vi "Test Initialization.vi"() -> ()   [LabVIEW 2020]
uses:
  Typedefs/FABR-Parameters.ctl
  Typedefs/FABR-Stimulus.ctl
  Typedefs/FABR-Sequence.ctl
  Typedefs/FABR-Order.ctl
  Typedefs/FABR-Response.ctl
  Typedefs/FABR-Runtime Data.ctl
  Typedefs/FABR-Stimulus Ticket.ctl
  Typedefs/FABR-Stimulus Condition.ctl
panel:
  out "resps":T1[](array[typedef])
  out "size(s)":i32
  out "stims":T1[](array[typedef])
  out "Tones":dbl[][](graph)
  out "SCL":cluster{T2[]}[](array[cluster])
  out "Runtime":T3
  in  "Params":T4={"Stimulus"={"Destination"="Speaker", "Rep rate (/sec)"=50.0, "Alternate Polarity"=FALSE, "Duration (ms)"=5.0, "Ramp (ms)"=0.5, "Fs (Hz)"=100000.0, "Frame size (s)"=1.0}, "Sequence"={"Freq"={"Start (kHz)"=0.25, "Stop (kHz)"=4.0, "Step (oct)"=1.0, "Skip (oct)"=2.0}, "Level"={"Start (dB)"=20, "Stop (dB)"=80, "Step (dB)"=10}, "Order"=enum."Interleaved"}, "Response"={"Gain"=1.0, "Averages"=0, "Window (ms)"=0.0, "Fs (Hz)"=25000.0}, "Reject"=0.0} {"Sequence"."Level"."Start (dB)" step=5; "Sequence"."Freq"."Start (kHz)" step=5.0; "Response"."Window (ms)" format="%.2f"}
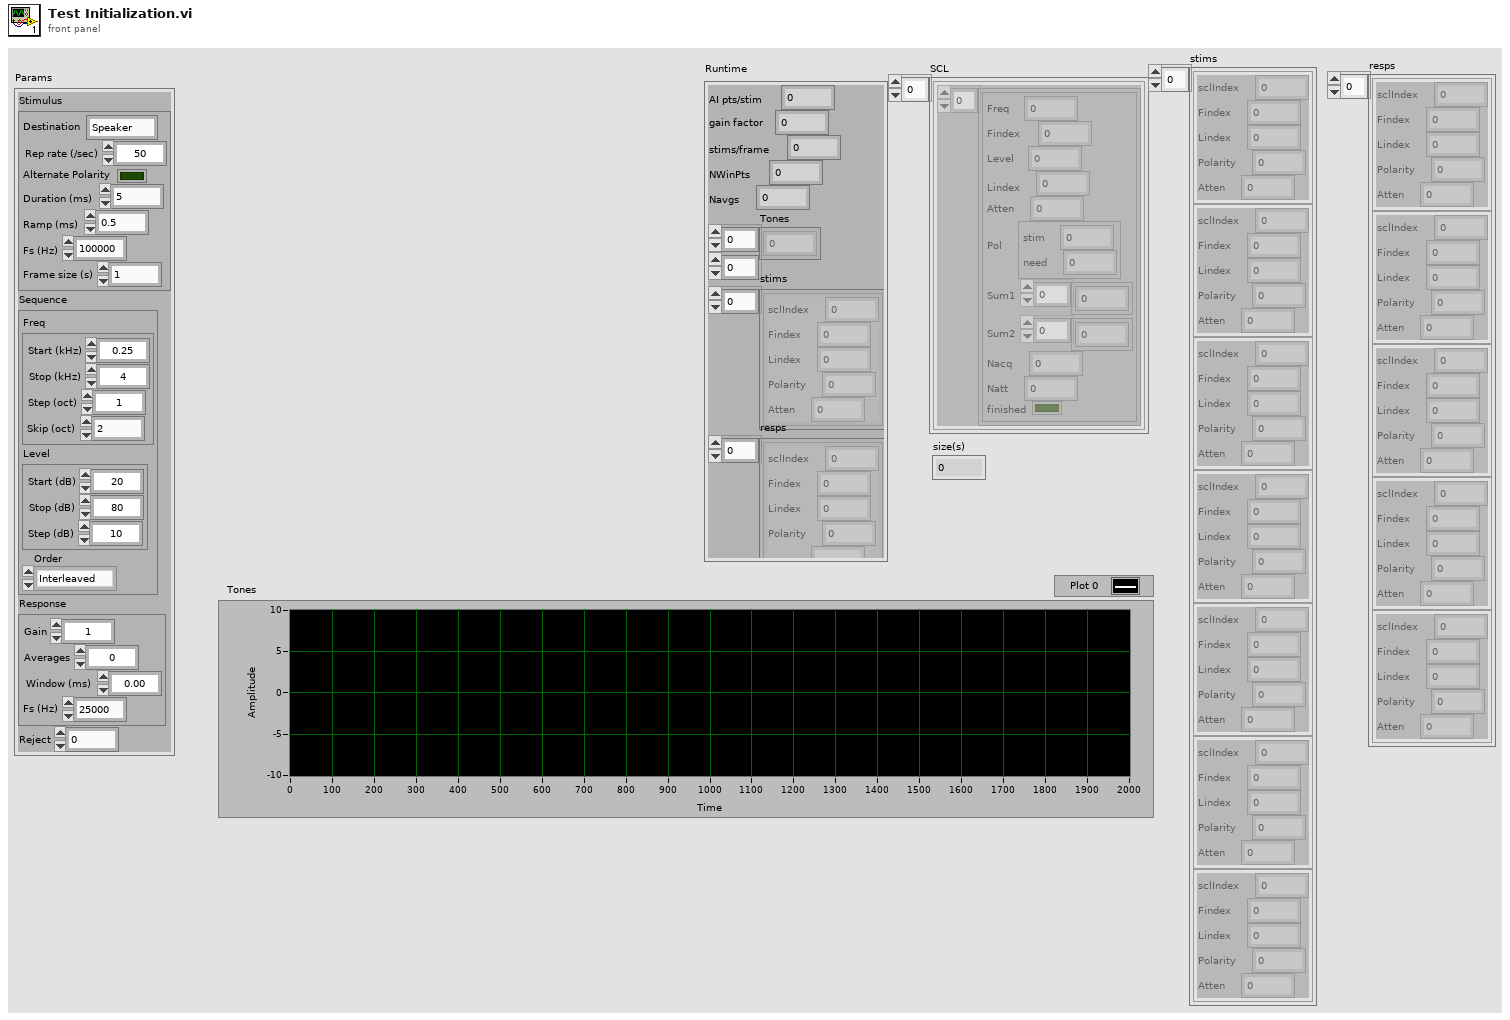
[diagram p1: front panel]
types:
  T1 = typedef "FABR-Stimulus Ticket.ctl" = cluster{"sclIndex":i32, "Findex":i32, "Lindex":i32, "Polarity":i32, "Atten":dbl}
  T2 = typedef "FABR-Stimulus Condition.ctl" = cluster{"Freq":dbl, "Findex":i32, "Level":dbl, "Lindex":i32, "Atten":dbl, "Pol":cluster{"stim":i32, "need":i32}, "Sum1":dbl[], "Sum2":dbl[], "Nacq":i32, "Natt":i32, "finished":bool}
  T3 = typedef "FABR-Runtime Data.ctl" = cluster{"AI pts/stim":i32, "gain factor":dbl, "stims/frame":i32, "NWinPts":i32, "Navgs":i32, "Tones":dbl[][], "stims":T1[], "resps":T1[]}
  T4 = typedef "FABR-Parameters.ctl" = cluster{"Stimulus":T5, "Sequence":T6, "Response":T8, "Reject":dbl}
  T5 = typedef "FABR-Stimulus.ctl" = cluster{"Destination":string, "Rep rate (/sec)":dbl, "Alternate Polarity":bool, "Duration (ms)":dbl, "Ramp (ms)":dbl, "Fs (Hz)":dbl, "Frame size (s)":dbl}
  T6 = typedef "FABR-Sequence.ctl" = cluster{"Freq":cluster{"Start (kHz)":dbl, "Stop (kHz)":dbl, "Step (oct)":dbl, "Skip (oct)":dbl}, "Level":cluster{"Start (dB)":i32, "Stop (dB)":i32, "Step (dB)":i32}, "Order":T7}
  T7 = typedef "FABR-Order.ctl" = enum16{"Interleaved"}
  T8 = typedef "FABR-Response.ctl" = cluster{"Gain":dbl, "Averages":i32, "Window (ms)":sgl, "Fs (Hz)":dbl}
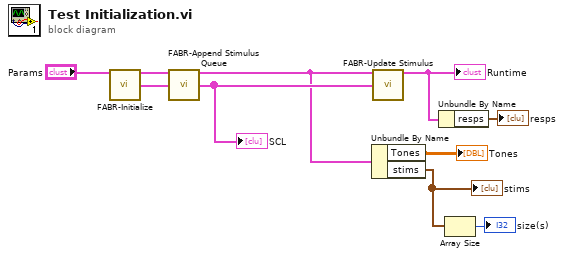
[diagram p0: block diagram]
diagram:
  n1 = call "FABR-Initialize.vi"("Params"="Params") -> ("Runtime"=w7:T3, "SCL"=w8:cluster{T2[]}[])  [unwired: 11 in, 2 out]
  n2 = call "FABR-Append Stimulus Queue.vi"("Runtime in"=w7, "SCL in"=w8) -> ("Runtime out"=w3:T3, "SCL thru"=w4:cluster{T2[]}[])  [unwired: 11 in, 1 out]
  "SCL" <- w4
  n3 = Unbundle By Name(w3) -> ("Tones"=→"Tones":dbl[][], "stims"=w6:T1[])
  "stims" <- w6
  n4 = call "FABR-Update Stimulus.vi"("Runtime in"=w3, "SCL in"=w4) -> ("Runtime out"=w2:T3)  [unwired: 11 in, 2 out]
  "Runtime" <- w2
  n5 = Unbundle By Name(w2) -> ("resps"=→"resps":T1[])
  n6 = Array Size(array=w6) -> (size(s)=→"size(s)":i32)
